vi "ZE_Recorder_ChoseTempChannelType.vi"(8 "error in":errorcluster, 11 "channel name":string="ss") -> (0 "error out":errorcluster, 3 "Cluster":T1={"ParameterBlock"=variant(cluster{"TC Type":u16, "TC Cold Junction":dbl, "Cold Junction Source":u16} {"TC Type"=10085, "TC Cold Junction"=25.0, "Cold Junction Source"=10200}), "TempChannelType"=enum."Thermocouple"})   [LabVIEW 2025, in "ZE_Recorder.lvlib"]
doc: "ZE_Recorder_ChoseTempChannelType.vi\n----------------------------------------------\n\n\nInputs:\n---------------------\n- error in : Cluster; \n- channel name : String; \n\nOutputs:\n---------------------\n- error out : Cluster; \n- Cluster : Cluster; \n\n----------------------------------------------\n22.05.2017\nZühlke Engineering AG\nCH-8952 Schlieren\nwww.zuehlke.com"
uses:
  ZE_Recorder.lvlib
  ZE_Recorder_TempType.ctl
  ZE_Recorder_TempParam.ctl
  ZE_Recorder_TempChannelAction.ctl
  ZE_Recorder_TCCluster.ctl
  ZE_Recorder_TCSource.ctl
  ZE_Recorder_TCType.ctl
  ZE_Recorder_RTDCluster.ctl
panel:
  in  "Cold Junction Source":u16(ring)=10200 items=["Built-In"=10200, "Constant Value"=10116]
  in  "RTD Iex":dbl=0.0005 min=1e-09 step=1e-05 format="%0.4f"
  in  "RTD Type":i32(ring)=10069 items=["Pt3750"=12481, "Pt3851"=10071, "Pt3911"=12482, "Pt3916"=10069, "Pt3920"=10053, "Pt3928"=12483, "Custom"=10137]
  in  "RTD Config":i32(ring)=2 items=["2-Wire"=2, "3-Wire"=3, "4-Wire"=4]
  out "Info":string="INFO: \nPlease use suitable NI hardware for RTD measurements. Parameter entry for custiom type follows in next step."
  in  "Config OK":bool
  in  "RTD R0":dbl=100.0 format="%0.2f"
  in  "TC Cold Junction":dbl=25.0 format="%0.2f"
  in  "TC Type":u16(ring)=10085 items=["J"=10072, "K"=10073, "N"=10077, "R"=10082, "S"=10085, "T"=10086, "B"=10047, "E"=10055]
  out "String":string="Chose your Sensor Type for Channel ss"
  in  "TempChannelType":T2
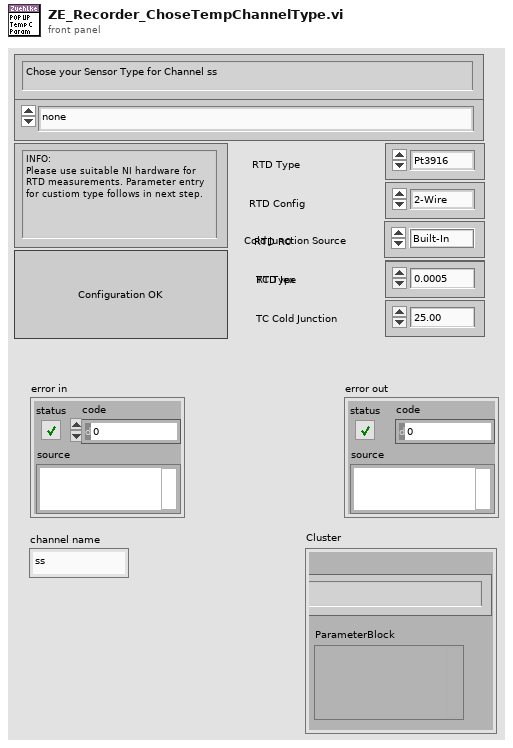
[diagram p1: front panel]
types:
  T1 = typedef "ZE_Recorder.lvlib/ZE_Recorder_TempParam.ctl" = cluster{"ParameterBlock":variant, "TempChannelType":T2}
  T2 = typedef "ZE_Recorder.lvlib/ZE_Recorder_TempType.ctl" = enum16{"none", "Thermocouple", "RTD", "Thermistor VE", "Thermistor CE"}
  T3 = typedef "ZE_Recorder.lvlib/ZE_Recorder_TempChannelAction.ctl" = enum16{"Get Channel Configs", "Read Config", "Add Config", "Clear"}
  T4 = typedef "ZE_Recorder.lvlib/ZE_Recorder_TCCluster.ctl" = cluster{"TC Cold Junction":dbl, "Cold Junction Source":T5, "TC Type":T6}
  T5 = typedef "ZE_Recorder.lvlib/ZE_Recorder_TCSource.ctl" = i32
  T6 = typedef "ZE_Recorder.lvlib/ZE_Recorder_TCType.ctl" = i32
  T7 = typedef "ZE_Recorder.lvlib/ZE_Recorder_RTDCluster.ctl" = cluster{"RTD R0":dbl, "RTD Iex":dbl, "RTD Type":i32, "RTD Config":i32}
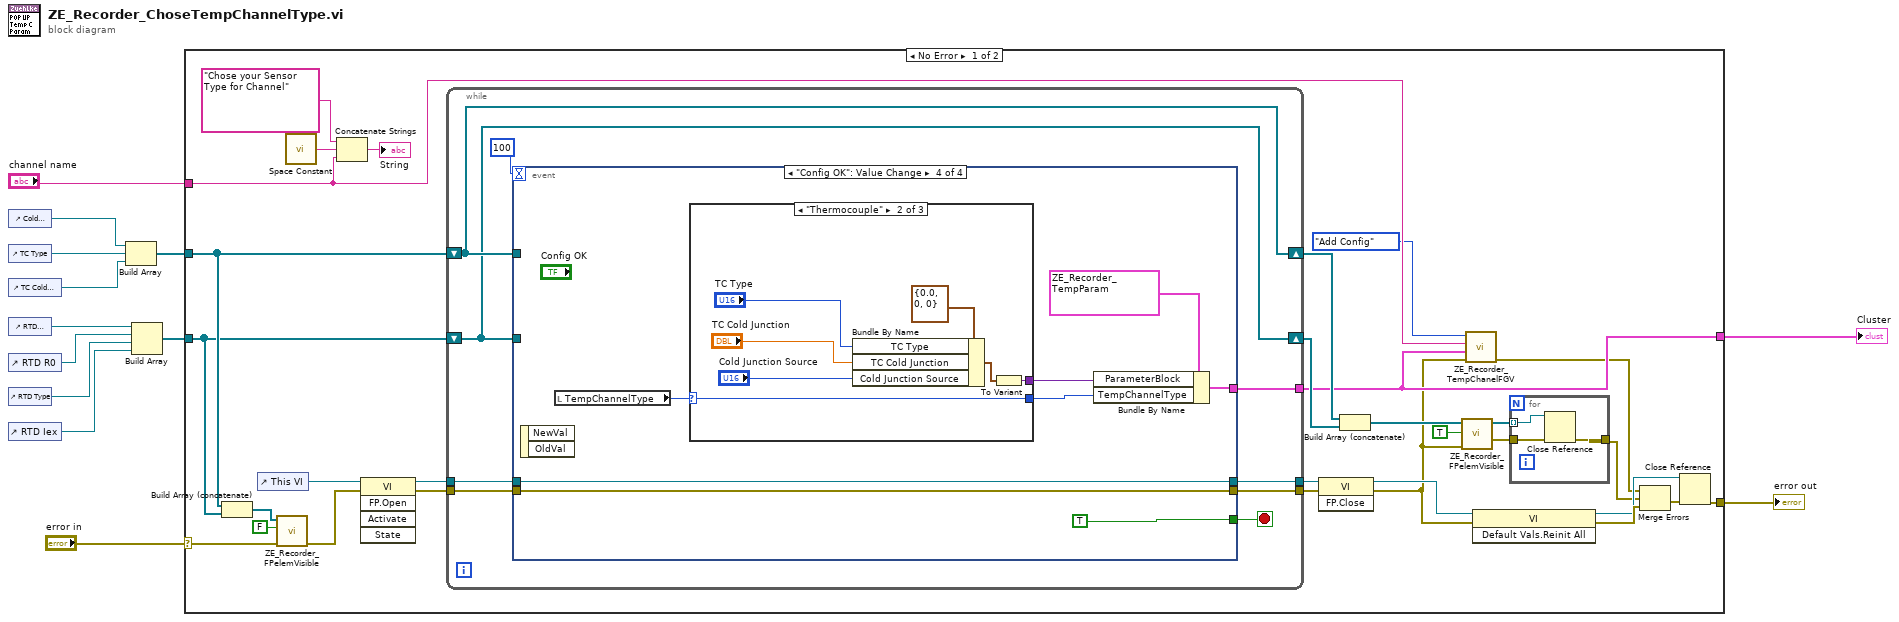
[diagram p0: block diagram]
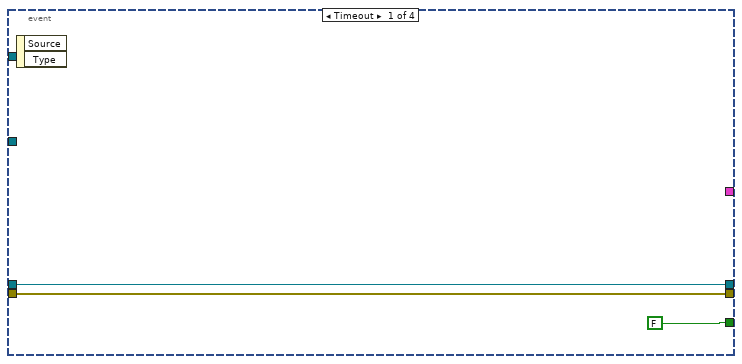
[diagram p2: hidden frame]
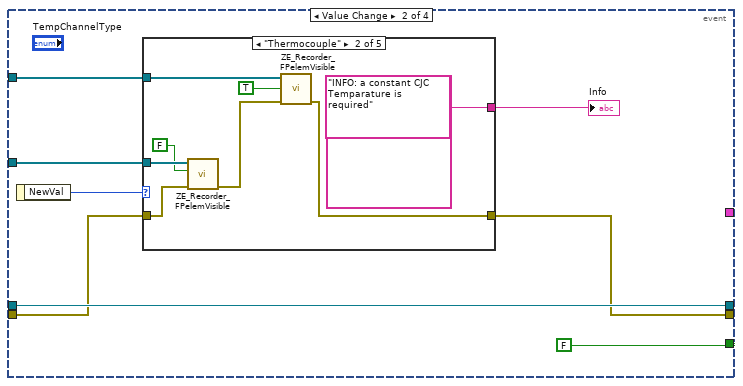
[diagram p3: hidden frame]
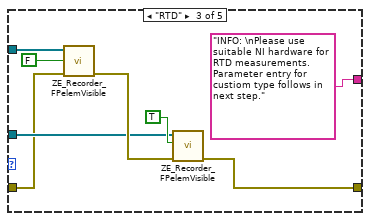
[diagram p5: hidden frame]
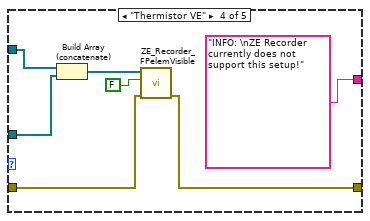
[diagram p6: hidden frame]
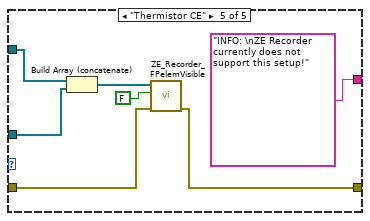
[diagram p7: hidden frame]
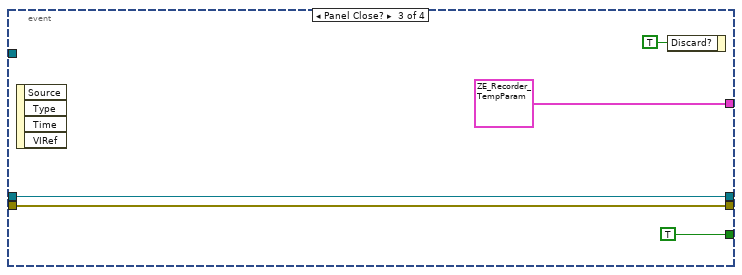
[diagram p8: hidden frame]
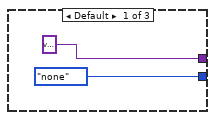
[diagram p9: hidden frame]
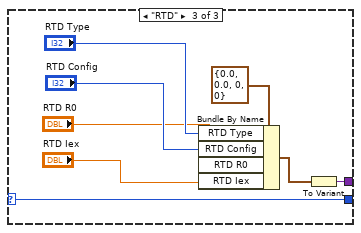
[diagram p10: hidden frame]
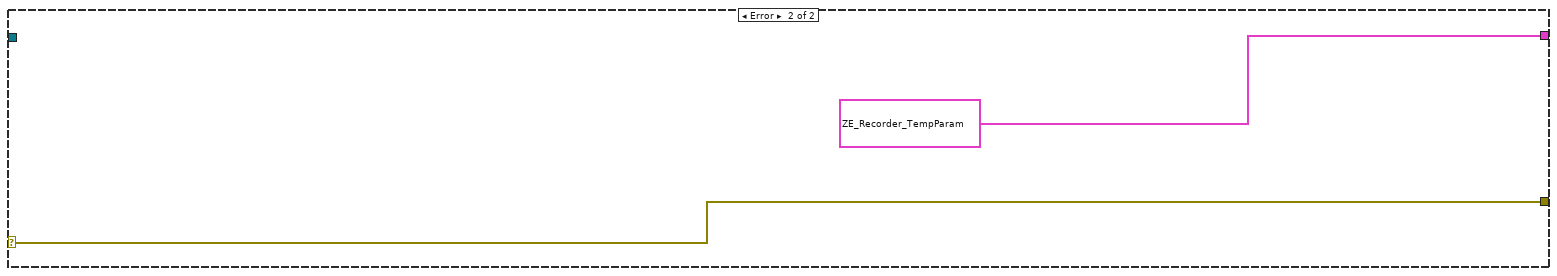
[diagram p11: hidden frame]
diagram:
  n1 = control-ref of="Cold Junction Source"() -> (w1:refnum<vi>)
  n2 = control-ref of="TC Type"() -> (w12:refnum<vi>)
  n3 = control-ref of="TC Cold Junction"() -> (w11:refnum<vi>)
  n4 = control-ref of="RTD Config"() -> (w3:refnum<vi>)
  n5 = control-ref of="RTD R0"() -> (w9:refnum<vi>)
  n6 = control-ref of="RTD Type"() -> (w4:refnum<vi>)
  n7 = control-ref of="RTD Iex"() -> (w2:refnum<vi>)
  n8 = Build Array(w1, w12, w11) -> (w10:refnum<vi>[])
  n9 = Build Array(w3, w9, w4, w2) -> (w8:refnum<vi>[])
  n10 = case shown="No Error" "error in" {
    selector: "error in" -> [w37 w129]
    tunnel: "channel name" -> [w18 _]
    tunnel: w10 -> [w35 _]
    tunnel: w8 -> [w34 _]
    tunnel: [w16 T1 {"ParameterBlock"=variant, "TempChannelType"=enum."Thermocouple"} ("Cluster 2")] -> w7
    tunnel: [w29 w129] -> w6
    frame No Error {
      n11 = Build Array (concatenate)(w35, w34) -> (w33:refnum<vi>[])
      n12 = control-ref of="This VI"() -> (w41:refnum<vi>)
      n13 = call "ZE_Recorder_FPelemVisible.vi"("error in"=w37, "Visible?"=FALSE, "FP Elems"=w33) -> ("error out"=w38:errorcluster)  [unwired: 7 in, 1 out]
      n14 = call <vilib>:"Space Constant.vi"() -> ("String"=w43:string)
      n15 = Concatenate Strings("Chose your Sensor Type for Channel", w43, w18) -> (→"String":string)
      n16 = invoke class="VI" method="FP.Open"(reference=w41, error in=w38) -> (reference out=w40:refnum<vi>, error out=w39:errorcluster)  [unwired: 3 in, 3 out]
      n17 = while {
        tunnel: w40 -> [w55]
        tunnel: w39 -> [w56]
        shift-right: [w53] -> w32
        shift-left: w35 -> [w53]
        shift-right: [w52] -> w31
        shift-left: w34 -> [w52]
        tunnel: [w51] -> w24
        tunnel: [w50] -> w30
        tunnel: [w49] -> w16
        stop <- w54 stop-if-true
        n18 = event shown="[3] \"Config OK\": Value Change" {
          selector: _ -> [_ _ _ _]
          dyn-events: _ -> [_ _ _ _]
          timeout: 100 -> [_ _ _ _]
          tunnel: w53 -> [_ w66 _ _]
          tunnel: w56 -> [w59 w64 w102 w108]
          tunnel: w55 -> [w58 w65 w101 w111]
          tunnel: [w58 w65 w101 w111] -> w50
          tunnel: w52 -> [_ w62 _ _]
          tunnel: [FALSE FALSE TRUE TRUE] -> w54
          tunnel: [w59 w61 w102 w108] -> w51
          tunnel: [_ _ T1 {"ParameterBlock"=variant, "TempChannelType"=enum."none"} ("Cluster 2") w106] -> w49
          event Timeout {
            n19 = event-data() -> ()  [unwired: 1 in, 2 out]
          }
          event Value Change {
            n20 = event-data() -> ("NewVal"=w67:T2)  [unwired: 1 in]
            n21 = case shown="\"Thermocouple\"" w67 {
              tunnel: w66 -> [_ w76 w82 w91 w94]
              tunnel: w64 -> [w68 w74 w79 w88 w96]
              tunnel: w62 -> [_ w72 w80 w90 w93]
              tunnel: [w68 w70 w78 w87 w95] -> w61
              tunnel: [_ "INFO: a constant CJC Temparature is required" ("Info 2") "INFO: \nPlease use suitable NI hardware for RTD measurements. Parameter entry for custiom type follows in next step." ("Info 2") "INFO: \nZE Recorder currently does not support this setup!" ("Info 2") "INFO: \nZE Recorder currently does not support this setup!" ("Info 2")] -> w60
              frame "none", Default {
              }
              frame "Thermocouple" {
                (unwired) "INFO: \nZE Recorder only supports setups with constant cold junction temparature!" ("Info 2")
                n22 = call "ZE_Recorder_FPelemVisible.vi"("error in"=w74, "Visible?"=FALSE, "FP Elems"=w72) -> ("error out"=w73:errorcluster)  [unwired: 7 in, 1 out]
                n23 = call "ZE_Recorder_FPelemVisible.vi"("error in"=w73, "Visible?"=TRUE ("Boolean"), "FP Elems"=w76) -> ("error out"=w70:errorcluster)  [unwired: 7 in, 1 out]
              }
              frame "RTD" {
                n24 = call "ZE_Recorder_FPelemVisible.vi"("error in"=w79, "Visible?"=FALSE ("Boolean"), "FP Elems"=w82) -> ("error out"=w81:errorcluster)  [unwired: 7 in, 1 out]
                n25 = call "ZE_Recorder_FPelemVisible.vi"("error in"=w81, "Visible?"=TRUE, "FP Elems"=w80) -> ("error out"=w78:errorcluster)  [unwired: 7 in, 1 out]
              }
              frame "Thermistor VE" {
                n26 = Build Array (concatenate)(w91, w90) -> (w89:refnum<vi>[])
                n27 = call "ZE_Recorder_FPelemVisible.vi"("error in"=w88, "Visible?"=FALSE, "FP Elems"=w89) -> ("error out"=w87:errorcluster)  [unwired: 7 in, 1 out]
              }
              frame "Thermistor CE" {
                n28 = Build Array (concatenate)(w94, w93) -> (w98:refnum<vi>[])
                n29 = call "ZE_Recorder_FPelemVisible.vi"("error in"=w96, "Visible?"=FALSE, "FP Elems"=w98) -> ("error out"=w95:errorcluster)  [unwired: 7 in, 1 out]
              }
            }
            "Info" <- w60
          }
          event Panel Close? {
            n30 = event-data() -> ()  [unwired: 1 in, 4 out]
            n31 = event-data("Discard?"=TRUE) -> ()  [unwired: 1 in, 1 out]
          }
          event "Config OK": Value Change {
            n32 = event-data() -> ()  [unwired: 1 in, 2 out]
            n33 = local read "TempChannelType"() -> (w109:T2)
            n34 = case shown="\"Thermocouple\"" w109 {
              selector: w109 -> [_ w120 w127]
              tunnel: [ZE_Recorder_TempType."none" ("TempChannelType") w120 w127] -> w105
              tunnel: [variant ("Variant") w119 w128] -> w104
              frame Default {
              }
              frame "Thermocouple" {
                n35 = Bundle By Name(cluster=T4 {"TC Cold Junction"=0.0, "Cold Junction Source"=0, "TC Type"=0} ("output cluster"), "TC Type"="TC Type", "TC Cold Junction"="TC Cold Junction", "Cold Junction Source"="Cold Junction Source") -> (w117:T4)
                n36 = To Variant(anything=w117) -> (Variant=w119:variant)
              }
              frame "RTD" {
                n37 = Bundle By Name(cluster=T7 {"RTD R0"=0.0, "RTD Iex"=0.0, "RTD Type"=0, "RTD Config"=0} ("output cluster"), "RTD Type"="RTD Type", "RTD Config"="RTD Config", "RTD R0"="RTD R0", "RTD Iex"="RTD Iex") -> (w121:T7)
                n38 = To Variant(anything=w121) -> (Variant=w128:variant)
              }
            }
            n39 = Bundle By Name(cluster=T1 {"ParameterBlock"=variant, "TempChannelType"=enum."Thermocouple"} ("Cluster 2"), "ParameterBlock"=w104, "TempChannelType"=w105) -> (w106:T1)
          }
        }
      }
      n40 = invoke class="VI" method="FP.Close"(reference=w30, error in=w24) -> (reference out=w23:refnum<vi>, error out=w15:errorcluster)  [unwired: 1 in, 1 out]
      n41 = Build Array (concatenate)(w32, w31) -> (w28:refnum<vi>[])
      n42 = call "ZE_Recorder_FPelemVisible.vi"("error in"=w15, "Visible?"=TRUE, "FP Elems"=w28) -> ("error out"=w26:errorcluster, "FP Elems out"=w27:refnum<vi>[])  [unwired: 7 in]
      n43 = call "ZE_Recorder_TempChanelFGV.vi"("error in"=w15, "Config In"=w16, "channel name in"=w18, "Action"=ZE_Recorder_TempChannelAction."Add Config") -> ("error out"=w14:errorcluster)  [unwired: 4 in, 3 out]
      n44 = invoke class="VI" method="Default Vals.Reinit All"(reference=w23, error in=w15) -> (reference out=w21:refnum<vi>, error out=w22:errorcluster)  [unwired: 1 in, 1 out]
      n45 = for {
        tunnel: w27 -> [w47] mode=indexing
        tunnel: w26 -> [w46]
        tunnel: [w45] -> w20
        n46 = Close Reference(reference=w47, error in (no error)=w46) -> (error out=w45:errorcluster)
      }
      n47 = Merge Errors(w14, w20, w22) -> (w19:errorcluster)
      n48 = Close Reference(reference=w21, error in (no error)=w19) -> (error out=w29:errorcluster)
    }
    frame Error {
    }
  }
  "Cluster" <- w7
  "error out" <- w6
